vi "Save as JUnit.vi"(8 "error in (no error)":errorcluster, 10 "Raw Results String":string, 11 "XML file path":path) -> (0 "error out":errorcluster, 2 "Test Header":T1={"name"="", "tests"=-1, "failures"=-1, "errors"=-1, "time"=-1.0, "disabled"=-1, "skipped"=-1, "skips"=-1, "timestamp"=-1.0, "hostname"="", "id"="", "package"="", "assertions"=-1, "file"="", "skip"="", "log"="", "url"=""})   [LabVIEW 2014, in "VI Tester Parsing.lvlib"]
uses:
  VI Tester Parsing.lvlib
  <vilib>/NI/JUnit Results API/Controls/Test Suite Attribute Values.ctl
  <vilib>/NI/JUnit Results API/Controls/Test Case Attributes.ctl
  <vilib>/NI/JUnit Results API/Controls/Outcome Attributes.ctl
  <vilib>/xml/Close Reference(Node).vi
  <vilib>/NI/JUnit Results API/JUnit API.lvlib
  <vilib>/xml/NI_XML.lvlib
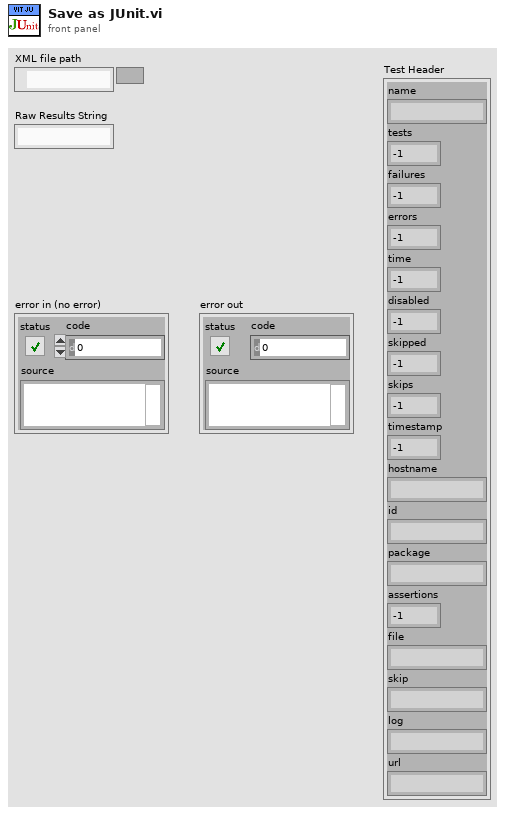
[diagram p1: front panel]
types:
  T1 = typedef "JUnit API.lvlib/Test Suite Attribute Values.ctl" = cluster{"name":string, "tests":i32, "failures":i32, "errors":i32, "time":dbl, "disabled":i32, "skipped":i32, "skips":i32, "timestamp":dbl, "hostname":string, "id":string, "package":string, "assertions":i32, "file":string, "skip":string, "log":string, "url":string}
  T2 = typedef "VI Tester Parsing.lvlib/Test Suite.ctl" = cluster{"Test Suite":string, "Tests":i32, "Failures":i32, "Errors":i32, "Time":dbl, "Test Cases":T3[]}
  T3 = typedef "VI Tester Parsing.lvlib/Test Case.ctl" = cluster{"Test Case":string, "Result":string, "Time":dbl, "Details":string}
  T4 = typedef "JUnit API.lvlib/Test Case Attributes.ctl" = cluster{"name":string, "assertions":i32, "time":dbl, "timestamp":dbl, "classname":string, "status":string, "class":string, "file":string, "line":string, "log":string, "group":string, "url":string}
  T5 = typedef "JUnit API.lvlib/Outcome Attributes.ctl" = cluster{"message":string, "type":string}
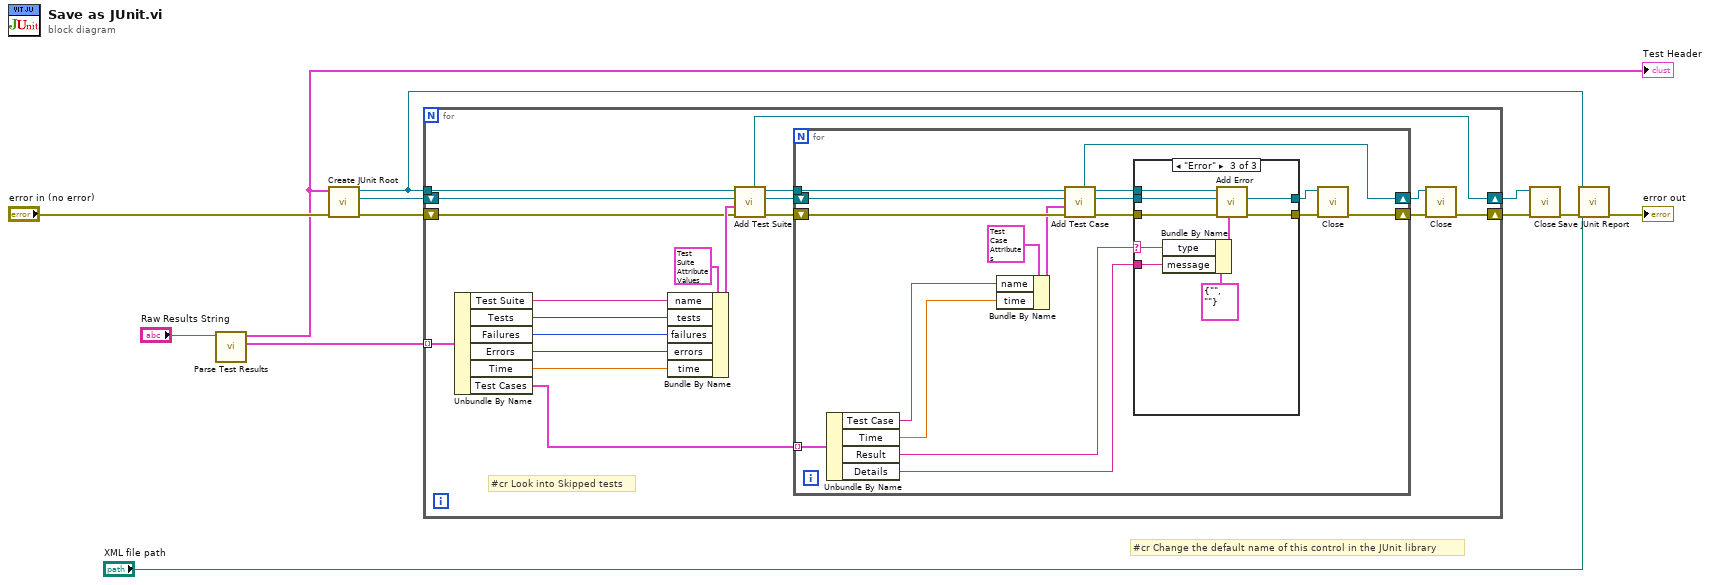
[diagram p0: block diagram]
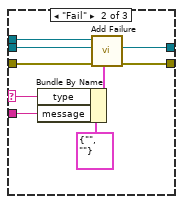
[diagram p3: hidden frame]
diagram:
  # "#cr Change the default name of this control in the JUnit library"
  n1 = call "Parse Test Results.vi"("Raw Test Results"="Raw Results String") -> ("Test Suites"=w3:T2[], "Test Header"=w2:T1)  [unwired: 9 in]
  "Test Header" <- w2
  n2 = call <vilib>:"Create JUnit Root.vi"("Error In (No Error)"="error in (no error)", "Test Suites Atrributes"=w2) -> ("Error Out"=w5:errorcluster, "Teststuites Ref"=w4:refnum<k20>, "File Ref Out"=w9:refnum<k20>)  [unwired: 7 in]
  n3 = for {
    tunnel: w3 -> [w29] mode=indexing
    shift-right: [w17] -> w7
    shift-left: w4 -> [w30]
    shift-right: [w16] -> w6
    shift-left: w5 -> [w24]
    tunnel: w9 -> [w31]
    # "#cr Look into Skipped tests"
    n4 = Unbundle By Name(w29) -> ("Test Suite"=w27:string, "Tests"=w26:i32, "Failures"=w15:i32, "Errors"=w13:i32, "Time"=w14:dbl, "Test Cases"=w20:T3[])
    n5 = Bundle By Name(cluster=T1 {"name"="", "tests"=-1, "failures"=-1, "errors"=-1, "time"=-1.0, "disabled"=-1, "skipped"=-1, "skips"=-1, "timestamp"=-1.0, "hostname"="", "id"="", "package"="", "assertions"=-1, "file"="", "skip"="", "log"="", "url"=""} ("Test Suite Atrributes"), "name"=w27, "tests"=w26, "failures"=w15, "errors"=w13, "time"=w14) -> (w25:T1)
    n6 = call <vilib>:"Add Test Suite.vi"("Error In (No Error)"=w24, "Test Suite Atrributes"=w25, "Teststuites Ref In"=w30, "File Ref In"=w31) -> ("Error Out"=w23:errorcluster, "Testsuite Ref"=w21:refnum<k20>, "File Ref Out"=w22:refnum<k20>, "Teststuites Ref Out"=w17:refnum<k20>)  [unwired: 4 in]
    n7 = for {
      shift-right: [w33] -> w18
      shift-left: w21 -> [w46]
      tunnel: w20 -> [w45] mode=indexing
      shift-right: [w32] -> w19
      shift-left: w23 -> [w48]
      tunnel: w22 -> [w47]
      n8 = Unbundle By Name(w45) -> ("Test Case"=w44:string, "Time"=w43:dbl, "Result"=w37:string, "Details"=w36:string)
      n9 = Bundle By Name(cluster=T4 {"name"="", "assertions"=-1, "time"=-1.0, "timestamp"=-1.0, "classname"="", "status"="", "class"="", "file"="", "line"="", "log"="", "group"="", "url"=""} ("Test Case Atrributes"), "name"=w44, "time"=w43) -> (w38:T4)
      n10 = call <vilib>:"Add Test Case.vi"("Error In (No Error)"=w48, "Test Case Atrributes"=w38, "Testsuite Ref In"=w46, "File Ref In"=w47) -> ("error out"=w40:errorcluster, "Testcase Ref"=w41:refnum<k20>, "File Ref Out"=w42:refnum<k20>, "Testsuite Ref Out"=w33:refnum<k20>)  [unwired: 4 in]
      n11 = case shown="\"Error\"" w37 {
        selector: w37 -> [_ w56 w68]
        tunnel: w42 -> [_ w59 w60]
        tunnel: w41 -> [w50 w58 w63]
        tunnel: w40 -> [w49 w57 w65]
        tunnel: w36 -> [_ w55 w67]
        tunnel: [w49 w54 w64] -> w35
        tunnel: [w50 w53 w62] -> w34
        frame "Pass", Default {
        }
        frame "Fail" {
          n12 = Bundle By Name(cluster=T5 {"message"="", "type"=""} ("Failure Attributes"), "type"=w56, "message"=w55) -> (w52:T5)
          n13 = call <vilib>:"Add Failure.vi"("Outcome Attributes"=w52, "Error In (No Error)"=w57, "Testcase Ref"=w58, "File Ref In"=w59) -> ("Error Out"=w54:errorcluster, "Testcase Ref Out"=w53:refnum<k20>)  [unwired: 5 in, 1 out]
        }
        frame "Error" {
          n14 = Bundle By Name(cluster=T5 {"message"="", "type"=""} ("Failure Attributes"), "type"=w68, "message"=w67) -> (w61:T5)
          n15 = call <vilib>:"Add Error.vi"("Outcome Attributes"=w61, "Error In (No Error)"=w65, "Testcase Ref"=w63, "File Ref In"=w60) -> ("Error Out"=w64:errorcluster, "Testcase Ref Out"=w62:refnum<k20>)  [unwired: 5 in, 1 out]
        }
      }
      n16 = call-poly <vilib>:"Close.vi"("error in (no error)"=w35, "node"=w34) -> ("error out"=w32:errorcluster)  [unwired: 7 in]
    }
    n17 = call-poly <vilib>:"Close.vi"("error in (no error)"=w19, "node"=w18) -> ("error out"=w16:errorcluster)  [unwired: 7 in]
  }
  n18 = call-poly <vilib>:"Close.vi"("error in (no error)"=w6, "node"=w7) -> ("error out"=w8:errorcluster)  [unwired: 7 in]
  n19 = call <vilib>:"Save JUnit Report.vi"("Error In (No Error)"=w8, "XML file path"="XML file path", "File Ref In"=w9) -> ("Error Out"=→"error out":errorcluster)  [unwired: 8 in]
